vi "SetPressure_v1.vi"(2 "Debug Mode":bool, 3 "Elapsed Time (s)":dbl, 4 "State":enum16{"Edit", "Start", "Run", "End", "Idle"}(ring), 5 "Argument List In":string[](array[string])) -> (0 "Status Out":string, 1 "Argument List Out":string[](array[string]))   [LabVIEW 2011]
panel:
  out "error out":errorcluster
  in  "Set Point":string(combo)="C"
  in  "P (Torr)":dbl=76.0
  in  "Cancel":bool
  in  "OK":bool
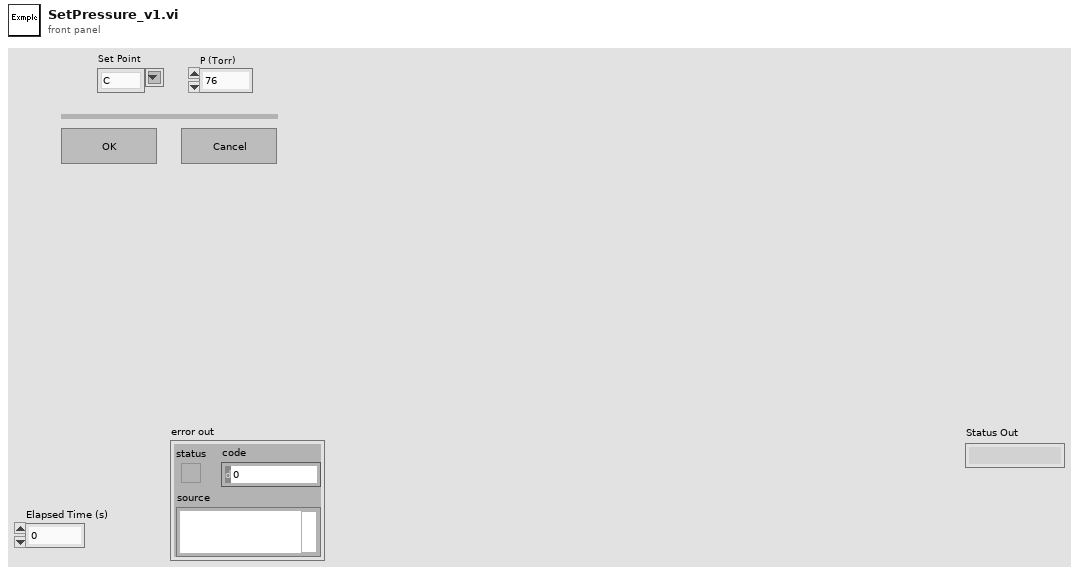
[diagram p1: front panel]
types:
  T1 = enum16{"Discrete", "Continuous", "Instantaneous"}
  T2 = enum32{"Invalid", "Default", "Floating", "Floating/Auto-Hide", "Modal"}
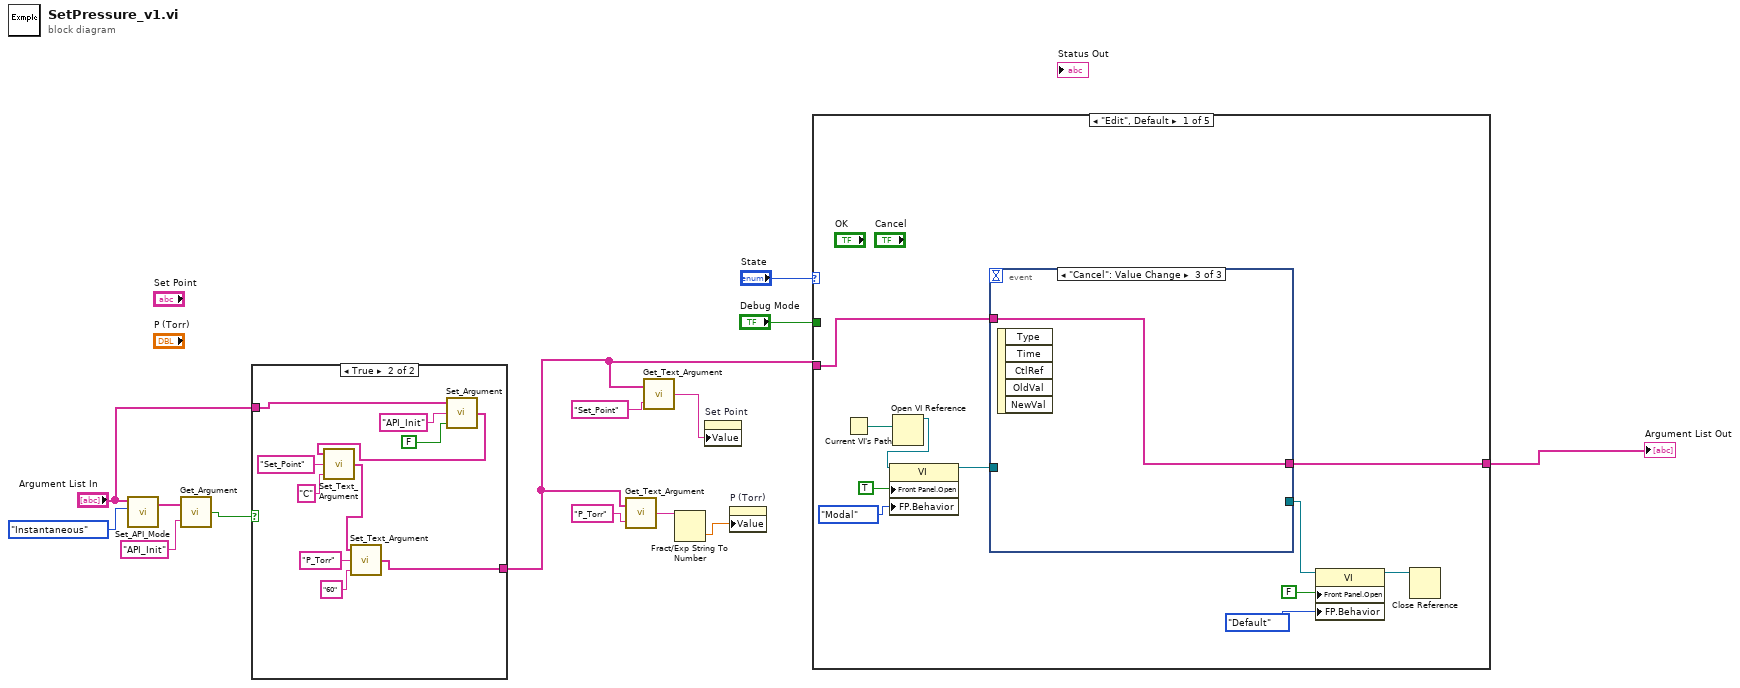
[diagram p0: block diagram]
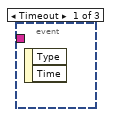
[diagram p3: hidden frame]
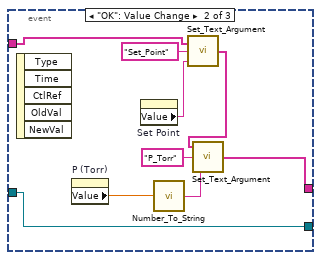
[diagram p4: hidden frame]
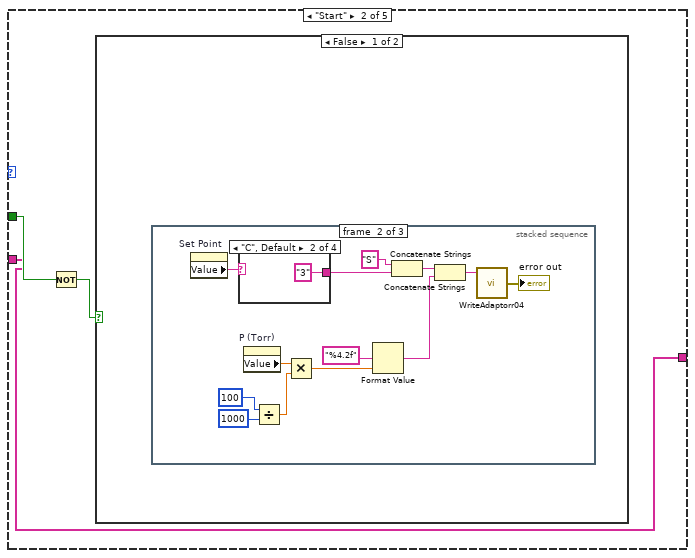
[diagram p5: hidden frame]
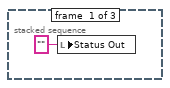
[diagram p6: hidden frame]
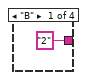
[diagram p7: hidden frame]
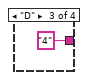
[diagram p8: hidden frame]
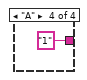
[diagram p9: hidden frame]
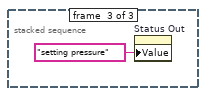
[diagram p10: hidden frame]
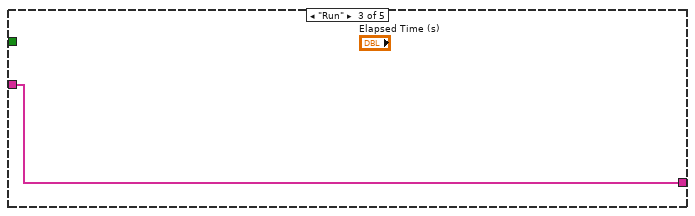
[diagram p12: hidden frame]
diagram:
  n1 = call "Set_API_Mode.vi"("API Mode"=T1."Instantaneous", "Argument List In"="Argument List In") -> ("Argument List Out"=w1:string[])  [unwired: 3 in]
  n2 = call "Get_Argument.vi"("Argument"="API_Init", "Argument List"=w1) -> ("Enabled"=w11:bool)
  n3 = case shown="True" w11 {
    tunnel: "Argument List In" -> [w15 w21]
    tunnel: [w15 w16] -> w5
    frame False {
    }
    frame True {
      n4 = call "Set_Argument.vi"("Enable"=FALSE, "Argument"="API_Init", "Argument List In"=w21) -> ("Argument List Out"=w20:string[])
      n5 = call "Set_Text_Argument.vi"("Text"="C", "Argument"="Set_Point", "Argument List In"=w20) -> ("Argument List Out"=w17:string[])
      n6 = call "Set_Text_Argument.vi"("Text"="60", "Argument"="P_Torr", "Argument List In"=w17) -> ("Argument List Out"=w16:string[])
    }
  }
  n7 = call "Get_Text_Argument.vi"("Argument"="P_Torr", "Argument List"=w5) -> ("Text"=w7:string)
  n8 = call "Get_Text_Argument.vi"("Argument"="Set_Point", "Argument List"=w5) -> ("Text"=w9:string)
  n9 = Fract/Exp String To Number(string=w7) -> (number=w6:dbl)  [unwired: 4 out]
  n10 = property on="Set Point" class="CmbBox"("Value"=w9) -> ()  [unwired: 2 in, 2 out]
  n11 = property on="P (Torr)" class="DigNum (strict)"("Value"=w6) -> ()  [unwired: 2 in, 2 out]
  n12 = case shown="\"Edit\", Default" "State" {
    tunnel: "Debug Mode" -> [_ w49 _ _ _]
    tunnel: w5 -> [w36 w47 w69 w70 w71]
    tunnel: [w35 w47 w69 w70 w71] -> w4
    frame "Edit", Default {
      n13 = Current VI's Path() -> (path=w33:path)
      n14 = Open VI Reference(vi path=w33) -> (vi reference=w32:refnum<vi>)  [unwired: 1 in, 5 out]
      n15 = property class="VI"(reference=w32, "Front Panel.Open"=TRUE ("Front Panel Window:Open"), "FP.Behavior"=T2."Modal" ("Front Panel Window:Behavior")) -> (reference out=w30:refnum<vi>)  [unwired: 1 in, 1 out]
      n16 = event shown="[2] \"Cancel\": Value Change" {
        selector: _ -> [_ _ _]
        dyn-events: _ -> [_ _ _]
        timeout: _ -> [_ _ _]
        tunnel: w36 -> [_ w40 w46]
        tunnel: [_ w38 w46] -> w35
        tunnel: w30 -> [_ w37 _]
        tunnel: [_ w37 _] -> w26
        event Timeout {
          n17 = event-data() -> ()  [unwired: 1 in, 2 out]
        }
        event "OK": Value Change {
          n18 = event-data() -> ()  [unwired: 1 in, 5 out]
          n19 = property on="P (Torr)" class="DigNum (strict)"() -> ("Value"=w43:dbl)  [unwired: 2 in, 2 out]
          n20 = property on="Set Point" class="CmbBox"() -> ("Value"=w44:string)  [unwired: 2 in, 2 out]
          n21 = call "Number_To_String.vi"("Number"=w43) -> ("String"=w41:string)
          n22 = call "Set_Text_Argument.vi"("Text"=w44, "Argument"="Set_Point", "Argument List In"=w40) -> ("Argument List Out"=w39:string[])
          n23 = call "Set_Text_Argument.vi"("Text"=w41, "Argument"="P_Torr", "Argument List In"=w39) -> ("Argument List Out"=w38:string[])
        }
        event "Cancel": Value Change {
          n24 = event-data() -> ()  [unwired: 1 in, 5 out]
        }
      }
      n25 = property class="VI"(reference=w26, "Front Panel.Open"=FALSE ("Front Panel Window:Open"), "FP.Behavior"=T2."Default" ("Front Panel Window:Behavior")) -> (reference out=w27:refnum<vi>)  [unwired: 1 in, 1 out]
      n26 = Close Reference(reference=w27) -> ()  [unwired: 1 in, 1 out]
    }
    frame "Start" {
      n27 = Not(x=w49) -> (.not. x?=w48:bool)
      n28 = case shown="False" w48 {
        frame False {
          n29 = stacked-sequence {
            frame #0 {
              n30 = local write "Status Out"("" ("Status Out")) -> ()
            }
            frame #1 {
              n31 = property on="Set Point" class="CmbBox"() -> ("Value"=w63:string)  [unwired: 2 in, 2 out]
              n32 = case shown="\"C\", Default" w63 {
                tunnel: ["2" "3" "4" "1"] -> w55
                frame "B" {
                }
                frame "C", Default {
                }
                frame "D" {
                }
                frame "A" {
                }
              }
              n33 = property on="P (Torr)" class="DigNum (strict)"() -> ("Value"=w52:dbl)  [unwired: 2 in, 2 out]
              n34 = Divide(x=100, y=1000) -> (x/y=w58:dbl)
              n35 = Multiply(x=w52, y=w58) -> (x*y=w61:dbl)
              n36 = Format Value(format string="%4.2f", value (0)=w61) -> (output string=w62:string)  [unwired: 1 in]
              n37 = Concatenate Strings("S", w55) -> (w53:string)
              n38 = Concatenate Strings(w53, w62) -> (w59:string)
              n39 = call "WriteAdaptorr04.vi"("string to write"=w59) -> ("error out"=→"error out":errorcluster)  [unwired: 2 in]
            }
            frame #2 {
              n40 = property on="Status Out" class="Str"("Value"="setting pressure" ("Status Out")) -> ()  [unwired: 2 in, 2 out]
            }
          }
        }
        frame True {
        }
      }
    }
    frame "Run" {
    }
    frame "End" {
    }
    frame "Idle" {
    }
  }
  "Argument List Out" <- w4
